vi "Monitor.vi"(8 "error in (no error)":errorcluster, 11 "PLC_Module in":refnum<class "PLC_Module.lvclass">) -> (0 "error out":errorcluster, 3 "PLC_Module out":refnum<class "PLC_Module.lvclass">)   [LabVIEW 2025, in "PLC_Module.lvlib" / "PLC_Module.lvclass"]
uses:
  PLC_Module.lvclass
  PLC_Module.lvclass/PLC_Module.ctl
  <vilib>/Utility/miscctls.llb/LVMapReplaceAction.ctl
  59c2ce60-2112-4573-bd3c-f0c6538ac243.vi
  Write Configuration.vi
  Read Configuration.vi
  Read Connect.vi
  <vilib>/JDP Science/JSONtext/Variant to JSON Text.vi
  <vilib>/JDP Science/JSONtext/LVClass Serializer/JSONtext LVClass Serializer.lvclass
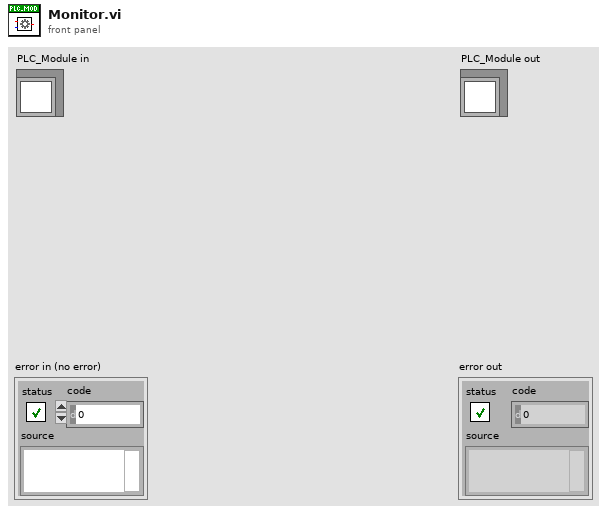
[diagram p1: front panel]
types:
  T1 = typedef "LVMapReplaceAction.ctl" = enum32{"Modify Entry only if found", "Add or Modify Entry", "Delete Entry"}
  T2 = typedef "PLC_Module.lvlib/PLC_Module.lvclass/PLC_Data_Config.ctl" = map{string, cluster{"Config":T3, "Get Value":string, "Set Value":string}}
  T3 = typedef "PLC_Module.lvlib/PLC_Module.lvclass/PLC_Data.ctl" = cluster{"Address":string, "Direction":enum16{"PC->PLC", "PLC->PC"}, "DataType":T4, "Description":string}
  T4 = typedef "PLC_Module.lvlib/PLC_Module.lvclass/PLC_Data_Type.ctl" = enum16{"Boolean", "Single Float", "U8", "U32", "U32_Array", "String"}
  T5 = cluster{"Config":T3, "Get Value":string, "Set Value":string}
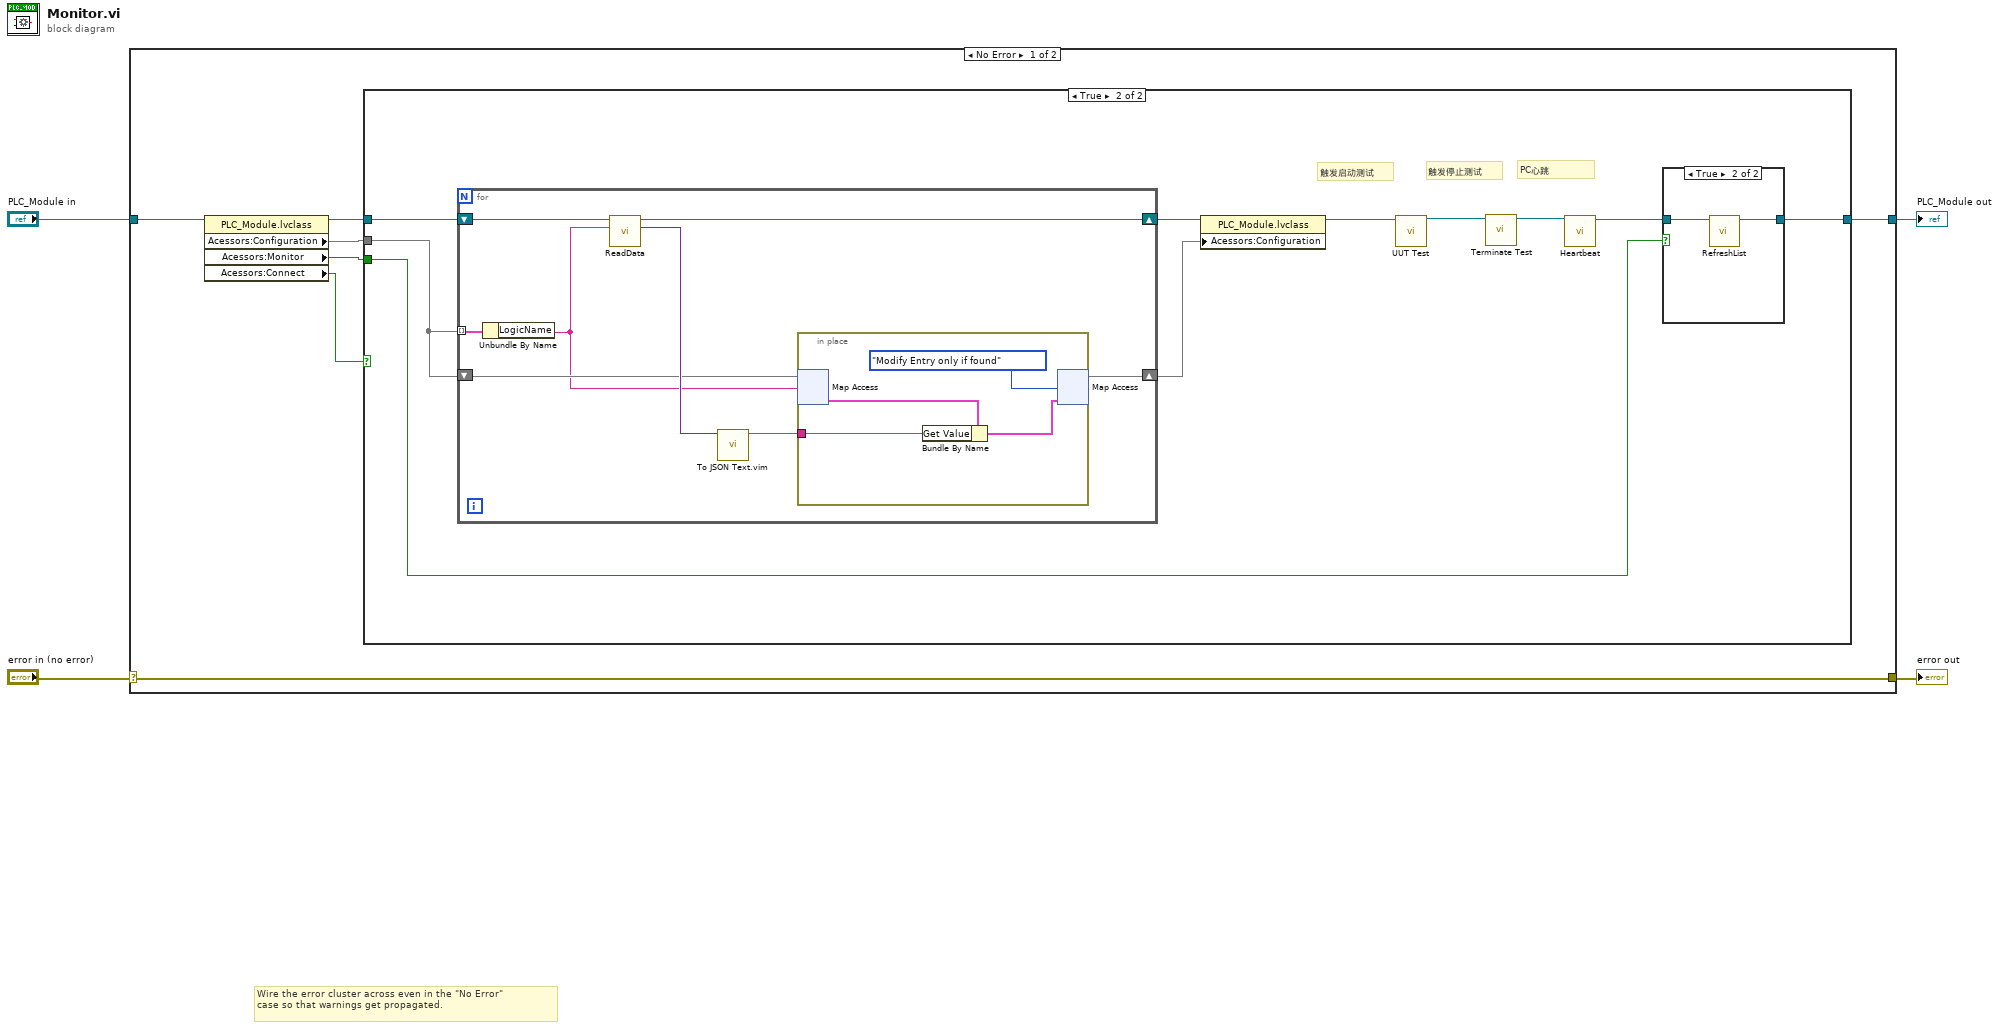
[diagram p0: block diagram]
diagram:
  # "Wire the error cluster across even in the \"No Error\"\ncase so that warnings get propagated."
  n1 = case shown="No Error" "error in (no error)" {
    selector: "error in (no error)" -> [w11 w39]
    tunnel: [w11 w39] -> w3
    tunnel: [w7 w38] -> w1
    tunnel: "PLC_Module in" -> [w10 w38]
    frame No Error {
      n2 = property class="PLC_Module.lvclass"(reference=w10) -> (reference out=w9:refnum<class "PLC_Module.lvclass">, "Acessors:Configuration"=w8:T2, "Acessors:Monitor"=w6:bool, "Acessors:Connect"=w5:bool)  [unwired: 1 in, 1 out]
      n3 = case shown="True" w5 {
        tunnel: w9 -> [w12 w21]
        tunnel: w8 -> [_ w20]
        tunnel: [w12 w18] -> w7
        tunnel: w6 -> [_ w17]
        frame False {
        }
        frame True {
          # "PC心跳"
          # "触发停止测试"
          # "触发启动测试"
          n4 = for {
            tunnel: w20 -> [w31] mode=indexing
            shift-right: [w32] -> w22
            shift-left: w21 -> [w33]
            shift-right: [w27] -> w19
            shift-left: w20 -> [w29]
            n5 = Unbundle By Name(w31) -> ("LogicName"=w28:string)
            n6 = call "ReadData.vi"("LogicName"=w28, "PLC_Module in"=w33) -> ("Data"=w30:variant, "PLC_Module out"=w32:refnum<class "PLC_Module.lvclass">)  [unwired: 7 in, 1 out]
            n7 = call "To JSON Text.vim"("Anything"=w30) -> ("<JSON>"=w26:string)  [unwired: 9 in, 1 out]
            n8 = in-place {
              in-place-border: w26 -> [w34]
              n9 = in-place-map #1(w29, w28) -> (w36:T5)  [unwired: 1 in, 1 out]
              n10 = Bundle By Name(cluster=w36, "Get Value"=w34) -> (w35:T5)
              n11 = in-place-map #1(w35, LVMapReplaceAction."Modify Entry only if found" ("action")) -> (w27:T2)  [unwired: 2 out]
            }
          }
          n12 = property class="PLC_Module.lvclass"(reference=w22, "Acessors:Configuration"=w19) -> (reference out=w16:refnum<class "PLC_Module.lvclass">)  [unwired: 1 in, 1 out]
          n13 = call "UUT Test.vi"("PLC_Module in"=w16) -> ("PLC_Module out"=w15:refnum<class "PLC_Module.lvclass">)  [unwired: 9 in, 1 out]
          n14 = call "Terminate Test.vi"("PLC_Module in"=w15) -> ("PLC_Module out"=w14:refnum<class "PLC_Module.lvclass">)  [unwired: 9 in, 1 out]
          n15 = call "Heartbeat.vi"("PLC_Module in"=w14) -> ("PLC_Module out"=w13:refnum<class "PLC_Module.lvclass">)  [unwired: 9 in, 1 out]
          n16 = case shown="True" w17 {
            tunnel: w13 -> [w23 w25]
            tunnel: [w23 w24] -> w18
            frame False {
            }
            frame True {
              n17 = call "RefreshList.vi"("PLC_Module in"=w25) -> ("PLC_Module out"=w24:refnum<class "PLC_Module.lvclass">)  [unwired: 9 in, 1 out]
            }
          }
        }
      }
    }
    frame Error {
    }
  }
  "error out" <- w3
  "PLC_Module out" <- w1
